vi "Add Database to SysDef.vi"(8 "error in":errorcluster, 10 "DB Alias":string="Diagnostics_Addon_Temp_DB", 11 "Item Ref in":T1 format="%.0x") -> (0 "error out":errorcluster, 3 "Item Ref out":T1 format="%.0x")   [LabVIEW 2025, in "Protection and Counter Addon Shared.lvlib"]
uses:
  Protection and Counter Addon Shared.lvlib
  <vilib>/NI/NI VeriStand Advanced SysDef API/SysDef API/Advanced System Definition.lvlib
  <vilib>/NI/NI VeriStand Advanced SysDef API/_SubVIs/SysDef.Property.Set.String.vi
  <vilib>/NI/NI VeriStand Advanced SysDef API/_SubVIs/SysDef.Search.Name.vi
  <vilib>/NI/NI VeriStand Advanced SysDef API/_SubVIs/SysDef.Search.GUID.vi
  <vilib>/NI/NI VeriStand Advanced SysDef API/_SubVIs/SysDef.Search.Target.vi
  <vilib>/NI VeriStand/Custom Device API/Custom Device Item Ref.ctl
  <vilib>/NI VeriStand/Custom Device API/Custom Device API.lvlib
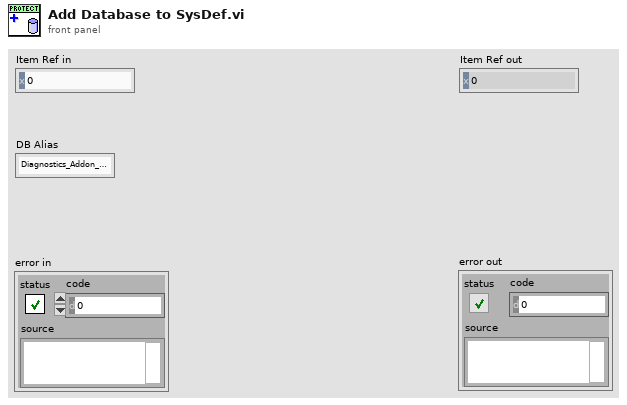
[diagram p1: front panel]
types:
  T1 = typedef "Custom Device API.lvlib/Custom Device Item Ref.ctl" = u64
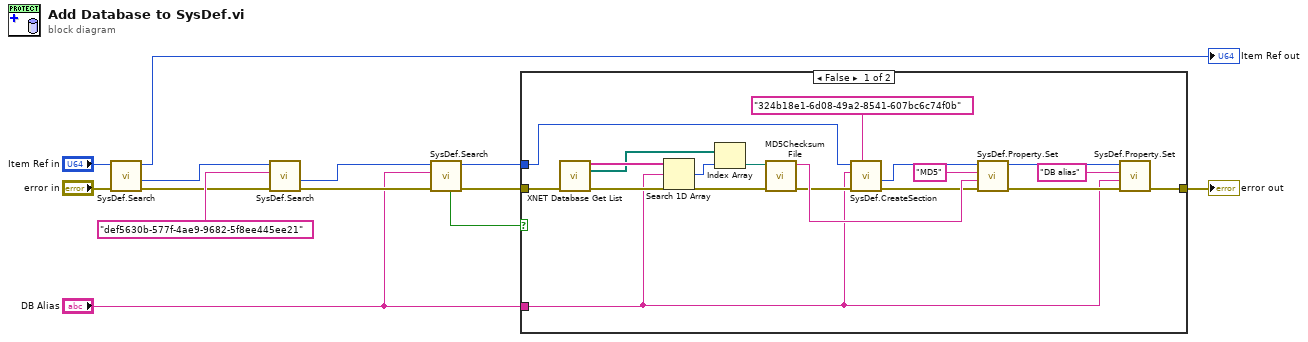
[diagram p0: block diagram]
diagram:
  n1 = call-poly <vilib>:"SysDef.Search.vi"("error in (no error)"="error in", "nodeID"="Item Ref in") -> ("error out"=w10:errorcluster, "Value out"=w9:u64, "nodeID out"=→"Item Ref out":u64)  [unwired: 6 in, 1 out]
  n2 = call-poly <vilib>:"SysDef.Search.vi"("error in (no error)"=w10, "GUID"="def5630b-577f-4ae9-9682-5f8ee445ee21" ("string"), "nodeID"=w9) -> ("error out"=w11:errorcluster, "Value out"=w12:u64)  [unwired: 5 in, 2 out]
  n3 = call-poly <vilib>:"SysDef.Search.vi"("error in (no error)"=w11, "Name"="DB Alias", "nodeID"=w12) -> ("error out"=w8:errorcluster, "nodeID out"=w7:u64, "Found?"=w6:bool)  [unwired: 5 in, 1 out]
  n4 = case shown="False" w6 {
    tunnel: [w22 w32] -> w5
    tunnel: w8 -> [w20 w32]
    tunnel: w7 -> [w21 _]
    tunnel: "DB Alias" -> [w14 _]
    frame False {
      n5 = call <vilib>:"XNET Database Get List.vi"("error in (no error)"=w20) -> ("array of alias"=w18:string[], "array of filepath"=w16:path[], "error out"=w19:errorcluster)  [unwired: 12 in]
      n6 = Search 1D Array(1D array=w18, element=w14) -> (index of element=w17:i32)  [unwired: 1 in]
      n7 = Index Array(array=w16, index=w17) -> (element=w15:path)
      n8 = call <vilib>:"MD5Checksum File.vi"("error in (no error)"=w19, "Path"=w15) -> ("error out"=w30:errorcluster, "MD5 message-digest"=w31:string)  [unwired: 8 in]
      n9 = call <vilib>:"SysDef.CreateSection.vi"("GUID"="324b18e1-6d08-49a2-8541-607bc6c74f0b" ("GUID (Default Section)"), "error in (no error)"=w30, "Name"=w14, "nodeID"=w21) -> ("error out"=w24:errorcluster, "New NodeID"=w23:u64)  [unwired: 4 in, 2 out]
      n10 = call-poly <vilib>:"SysDef.Property.Set.vi"("error in (no error)"=w24, "Value"=w31, "Property Name"="MD5", "nodeID"=w23) -> ("error out"=w25:errorcluster, "nodeID out"=w26:u64)  [unwired: 6 in]
      n11 = call-poly <vilib>:"SysDef.Property.Set.vi"("error in (no error)"=w25, "Value"=w14, "Property Name"="DB alias", "nodeID"=w26) -> ("error out"=w22:errorcluster)  [unwired: 6 in, 1 out]
    }
    frame True {
    }
  }
  "error out" <- w5
